vi "H.Signal.vi"() -> (2 "element":bool, 4 "Slide servo home RS":bool, 6 "HI Bit Auto":bool, 10 "Error Message":string, 14 "Message":string, 15 "Bool_H Sig":bool)   [LabVIEW 2015]
uses:
  Galobal variable_TI.vi
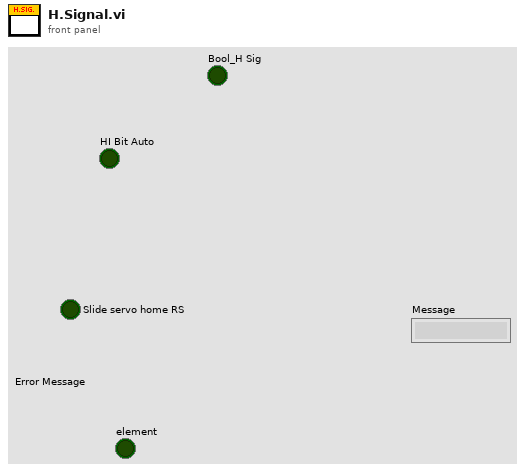
[diagram p1: front panel]
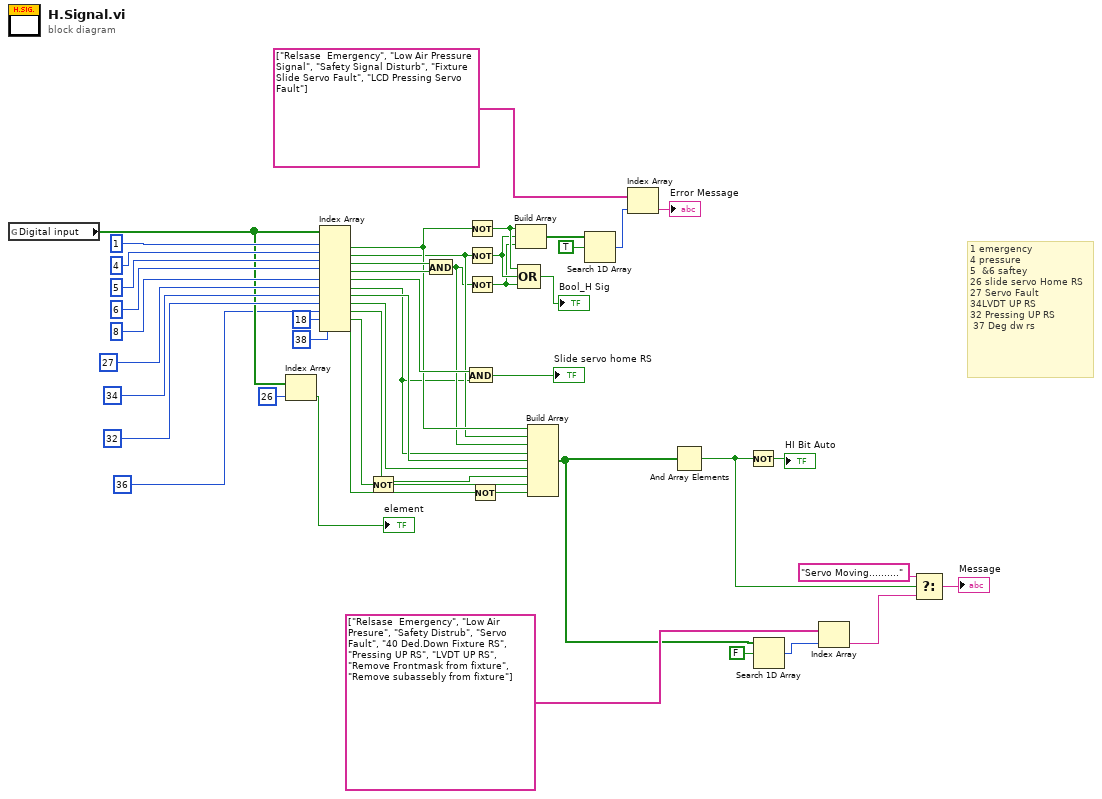
[diagram p0: block diagram]
diagram:
  # "1 emergency\n4 pressure\n5  &6 saftey\n26 slide servo Home RS\n27 Servo Fault\n34LVDT UP RS\n32 Pressing UP RS \n 37 Deg dw rs"
  n1 = global read "Galobal variable_TI.vi" "Digital input"() -> (w21:bool[])
  n2 = Index Array(array=w21, index=26) -> (element=→"element":bool)
  n3 = Index Array(array=w21, index #1=1 ("index"), index #2=4 ("index"), index #3=5 ("index"), index #4=6 ("index"), index #5=8 ("index"), index #6=27 ("index"), index #7=34 ("index"), index #8=32 ("index"), index #9=36 ("index"), index #10=18 ("index"), index #11=38 ("index")) -> (element #1=w28:bool, element #2=w27:bool, element #3=w42:bool, element #4=w41:bool, element #5=w30:bool, element #6=w16:bool, element #7=w24:bool, element #8=w22:bool, element #9=w17:bool, element #10=w6:bool, element #11=w5:bool)
  n4 = Not(x=w6) -> (.not. x?=w4:bool)
  n5 = And(x=w42, y=w41) -> (x .and. y?=w26:bool)
  n6 = And(x=w30, y=w16) -> (x .and. y?=→"Slide servo home RS":bool)
  n7 = Not(x=w28) -> (.not. x?=w34:bool)
  n8 = Not(x=w27) -> (.not. x?=w33:bool)
  n9 = Not(x=w26) -> (.not. x?=w32:bool)
  n10 = Not(x=w5) -> (.not. x?=w3:bool)
  n11 = Build Array(w34, w33, w32) -> (w37:bool[])
  n12 = Compound Arithmetic op=OR(w34, w33, w32) -> (→"Bool_H Sig":bool)
  n13 = Build Array(w28, w27, w26, w16, w24, w22, w17, w4, w3) -> (w10:bool[])
  n14 = Search 1D Array(1D array=w37, element=TRUE) -> (index of element=w39:i32)  [unwired: 1 in]
  n15 = Index Array(array=string[] ["Relsase  Emergency", "Low Air Pressure Signal", "Safety Signal Disturb", "Fixture Slide Servo Fault", "LCD Pressing Servo Fault"], index=w39) -> (element=→"Error Message":string)
  n16 = And Array Elements(Boolean array=w10) -> (logical AND=w9:bool)
  n17 = Not(x=w9) -> (.not. x?=→"HI Bit Auto":bool)
  n18 = Search 1D Array(1D array=w10, element=FALSE) -> (index of element=w13:i32)  [unwired: 1 in]
  n19 = Index Array(array=string[] ["Relsase  Emergency", "Low Air Presure", "Safety Distrub", "Servo Fault", "40 Ded.Down Fixture RS", "Pressing UP RS", "LVDT UP RS", "Remove Frontmask from fixture", "Remove subassebly from fixture"], index=w13) -> (element=w12:string)
  n20 = Select(t="Servo Moving..........", s=w9, f=w12) -> (s? t:f=→"Message":string)
